vi "Initiate.vi"(8 "error in (no error)":errorcluster, 11 "Tektronix DPO MSO 2000 4000 in":refnum<class "Tektronix DPO MSO 2000 4000.lvclass">) -> (0 "error out":errorcluster, 3 "Tektronix DPO MSO 2000 4000 out":refnum<class "Tektronix DPO MSO 2000 4000.lvclass">)   [LabVIEW 2020, in "Tektronix DPO MSO 2000 4000.lvclass"]
uses:
  Tektronix DPO MSO 2000 4000.lvclass
  C:/Sandbox/Git_Sandbox/WiSpry Test Framework source code (LV20)/WiSpry Test Framework/Instruments/Instrument.lvclass
  Instrument.lvclass/Instrument.ctl
  Instrument.lvclass
  <instrlib>/Tektronix DPO MSO 2000 4000 Series/Tektronix DPO MSO 2000 4000 Series.lvlib
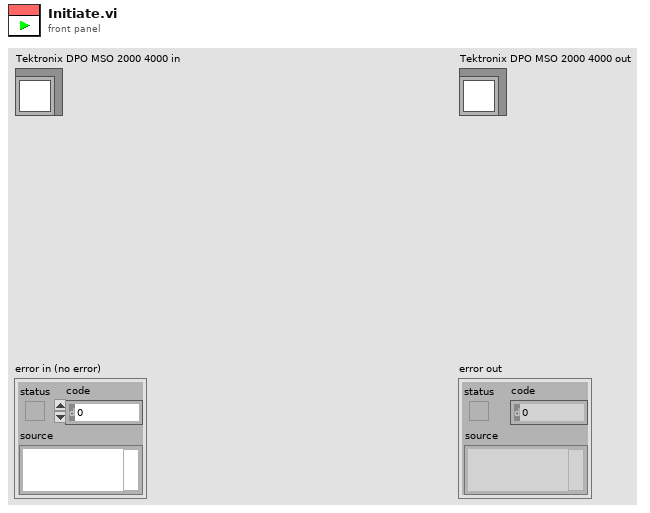
[diagram p1: front panel]
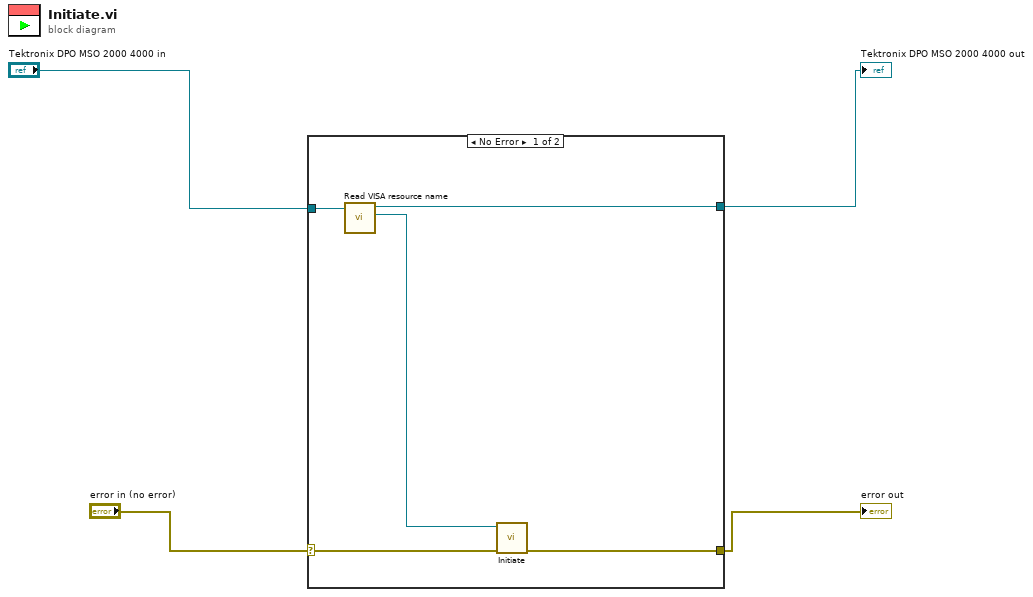
[diagram p0: block diagram]
diagram:
  n1 = case shown="No Error" "error in (no error)" {
    selector: "error in (no error)" -> [w8 w10]
    tunnel: [w5 w11] -> w1
    tunnel: "Tektronix DPO MSO 2000 4000 in" -> [w9 w11]
    tunnel: [w7 w10] -> w2
    frame No Error {
      n2 = call "Read VISA resource name.vi"("Instrument in"=w9) -> ("VISA resource name"=w6:refnum<visa-resource-name>, "Instrument out"=w5:refnum<class "Tektronix DPO MSO 2000 4000.lvclass">)  [unwired: 9 in]
      n3 = call <instrlib>:"Initiate.vi"("error in (no error)"=w8, "VISA resource name"=w6) -> ("error out"=w7:errorcluster)  [unwired: 8 in, 1 out]
    }
    frame Error {
    }
  }
  "error out" <- w2
  "Tektronix DPO MSO 2000 4000 out" <- w1
